vi "Draw Named Glyph.vi"(4 "Size":dbl=16.0, 5 "Transform (Center)":refnum<class "Transform.lvclass">, 6 "Colors":T1={"Front"={"Color"=0, "Alpha"=255}, "Back"={"Color"=16448250, "Alpha"=255}}, 7 "Glyph Source in":refnum<class "Glyph Source.lvclass">, 8 "error in (no error)":errorcluster, 9 "Destination":refnum<class "Glyph Canvas.lvclass">, 10 "Glyph Name":string, 11 "Glyph Drawer in":refnum<class "Glyph Drawer.lvclass">) -> (0 "error out":errorcluster, 1 "Destination Out":refnum<class "Glyph Canvas.lvclass">, 3 "Glyph Drawer out":refnum<class "Glyph Drawer.lvclass">)   [LabVIEW 2023, in "Font Glyph Drawer Interface.lvlib" / "Glyph Drawer.lvclass"]
uses:
  Glyph Drawer.lvclass
  Glyph Source/Glyph Source.lvclass
  Glyph Canvas/Glyph Canvas.lvclass
  Transform/Transform.lvclass
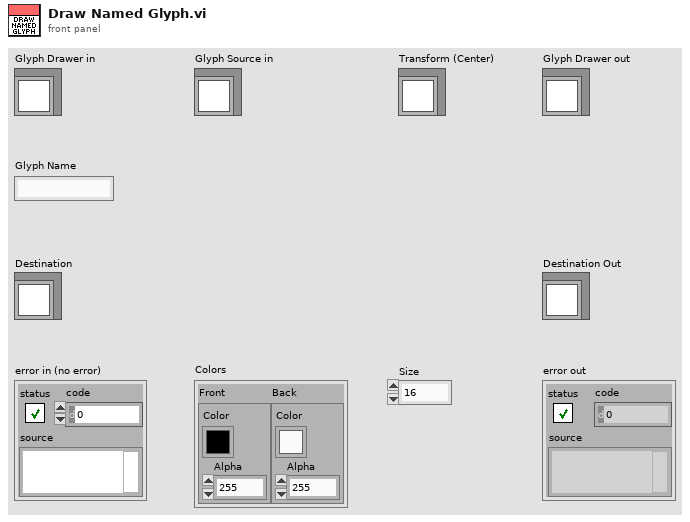
[diagram p1: front panel]
types:
  T1 = cluster{"Front":cluster{"Color":u32, "Alpha":u8}, "Back":cluster{"Color":u32, "Alpha":u8}}
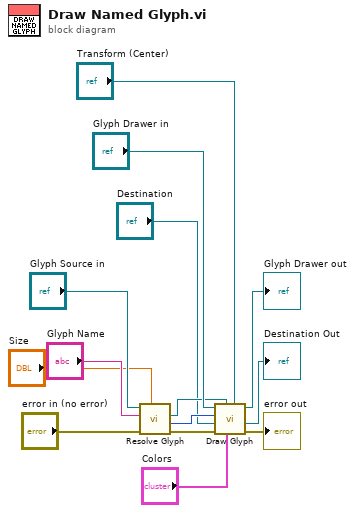
[diagram p0: block diagram]
diagram:
  n1 = call-dynamic "Resolve Glyph.vi"("Size"="Size", "error in (no error)"="error in (no error)", "Glyph Name"="Glyph Name", "Glyph Source in"="Glyph Source in") -> ("error out"=w10:errorcluster, "charcode"=w6:u32, "Font"=w7:refnum<class "Font Settings.lvclass">)  [unwired: 4 in, 1 out]
  n2 = call-dynamic "Draw Glyph.vi"("Transform (Center)"="Transform (Center)", "Colors"="Colors", "Font (System)"=w7, "error in (no error)"=w10, "Destination"="Destination", "codepoint"=w6, "Glyph Drawer in"="Glyph Drawer in") -> ("error out"=→"error out":errorcluster, "Destination Out"=→"Destination Out":refnum<class "Glyph Canvas.lvclass">, "Glyph Drawer out"=→"Glyph Drawer out":refnum<class "Glyph Drawer.lvclass">)  [unwired: 2 in]
